vi "SP_Final.vi"(1 "Table W/ Cmds":string[](array[string]), 2 "Commands Out":string[](array[string])) -> (0 "spreadsheet string":string)   [LabVIEW 2009]
panel:
  # "This LabVIEW item is deprecated.\n\nIt is believed to be unused and will be removed in a future version of SRV."
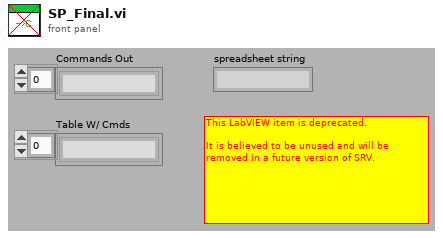
[diagram p1: front panel]
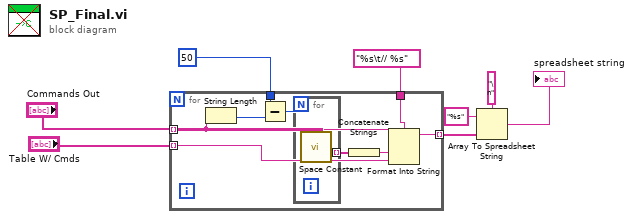
[diagram p0: block diagram]
diagram:
  n1 = for {
    tunnel: "Commands Out" -> [w12] mode=indexing
    tunnel: "Table W/ Cmds" -> [w17] mode=indexing
    tunnel: [w16] -> w8 mode=indexing
    tunnel: "%s\t// %s" ("format string") -> [w15]
    tunnel: 50 -> [w13]
    n2 = String Length(string=w12) -> (length=w14:i32)
    n3 = Subtract(x=w13, y=w14) -> (x-y=w11:i32)
    n4 = for {
      N: w11 -> [_]
      tunnel: [w18] -> w10 mode=indexing
      n5 = call <vilib>:"Space Constant.vi"() -> ("String"=w18:string)
    }
    n6 = Concatenate Strings(w10) -> (w9:string)
    n7 = Format Into String(format string=w15, initial string=w12, w9, w17) -> (resulting string=w16:string)  [unwired: 1 in, 1 out]
  }
  n8 = Array To Spreadsheet String(delimiter (Tab)="\n", array=w8, 3:"%s" ("format string")) -> (spreadsheet string=→"spreadsheet string":string)
